vi "Synchronized Acquisition.vi"() -> ()   [LabVIEW 2018, in "GettingStarted_5775_Host.lvlib"]
uses:
  GettingStarted_5775_Host.lvlib
  <vilib>/userDefined/High Color/nirio_resource_hc.ctl
  <instrlib>/FlexRIO/API/Host/v1/NI FlexRIO/API/Reference Clock Source.ctl
  <vilib>/FPGAPlugInAG/Dynamic/niLvFpga_Reset_Dynamic.vi
  <vilib>/FPGAPlugInAG/Dynamic/niLvFpga_Run_Dynamic.vi
  <instrlib>/FlexRIO/API/Host/v1/NI FlexRIO/API/Configure Reference Clock.vi
  <instrlib>/FlexRIO/API/Host/v1/NI FlexRIO/API/Configure Immediate Start Trigger.vi
  <instrlib>/FlexRIO/API/Host/v1/NI FlexRIO/API/Configure Analog Start Trigger.vi
  <instrlib>/FlexRIO/API/Host/v1/NI FlexRIO/API/Configure Digital Edge Start Trigger.vi
  <instrlib>/FlexRIO/API/Host/v1/NI FlexRIO/API/Get Property Reference - Fpga Small.vi
  <instrlib>/FlexRIO/API/Host/v1/NI FlexRIO/API/Read Stream 1D WDT.vi
  <vilib>/FPGAPlugInAG/Dynamic/niLvFpga_Close_Dynamic.vi
  <vilib>/rvi/interface/nirviMethod/nirviMethod.xnode
  <vilib>/rvi/interface/nirviCloseFPGA/nirviCloseFPGA.xnode
  <instrlib>/FlexRIO/API/Host/v1/NI FlexRIO API v1.lvlib
  <resource>/objmgr/sessionReference.rc
  <resource>/objmgr/niflexrioapiStream.rc
panel:
  in  "reference clock source":T1 items=["Default", "Onboard", "PXI_Clk10", "External", "None", "Baseboard Reference"]
  in  "stop":bool
  out "error out":errorcluster
  out "Waveform Graph":waveform(dbl)[](graph)
  in  "acquire pretrigger \nsamples?":bool
  in  "min. TClk period":dbl=1e-06 format="%#_6p"
  in  "trigger master index":i32
  in  "Tab Control":enum32{"Immediate", "Digital", "Analog"}(tab)
  in  "trigger source":string(combo)="PXI_Trig0"
  in  "rising edge?":bool=TRUE
  in  "trigger channel":string="AI0"
  in  "level (V)":dbl
  in  "hysteresis (V)":dbl
  in  "device configuration":T3(array[cluster])=[{"FlexRIO digitizer"="RIO0", "channels"="AI0", "samples"=65536, "bitfile path"=path ""}, {"FlexRIO digitizer"="RIO1", "channels"="AI0", "samples"=65536, "bitfile path"=path ""}]
  # "Overview: Configure multiple FlexRIO targets for a synchronized acquisition using the FlexRIO Host API and NI-TClk API.\nRequirements: FlexRIO, NI-TClk\nInstructions: \n 1. Fill in the device configuration array with the resource name of the FlexRIO digitizers to synchronize, as well as the number of samples and which channels to acquire on.\n 2. Specify which device should be used as the trigger master using trigger master index\n 3. Configure the trigger settings for the master device\n 4. Optionally configure the reference clock to be used\n 5. Run the VI"
  # "Trigger Master Configuration"
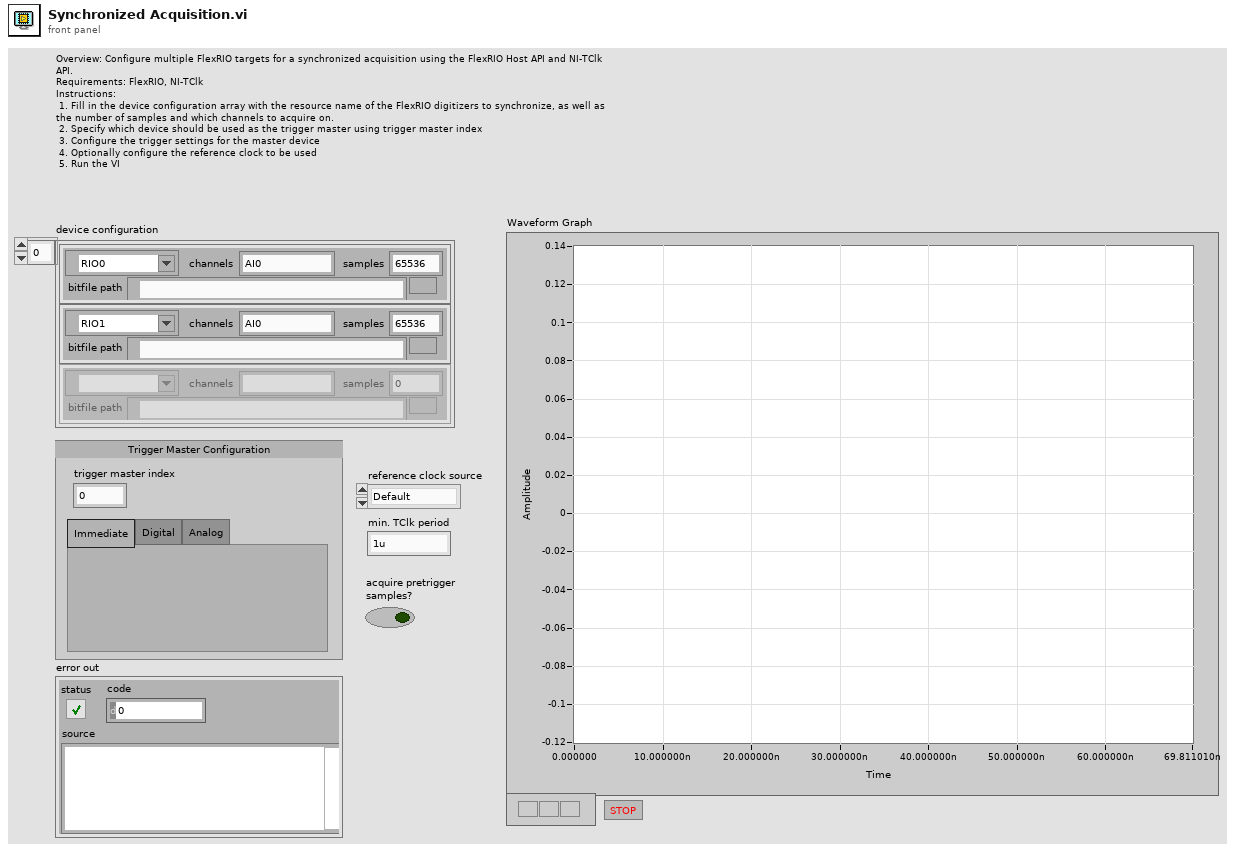
[diagram p1: front panel]
types:
  T1 = typedef "NI FlexRIO API v1.lvlib/Reference Clock Source.ctl" = i32
  T2 = typedef "nirio_resource_hc.ctl" = tag
  T3 = cluster{"FlexRIO digitizer":T2, "channels":string, "samples":u64, "bitfile path":path}[]
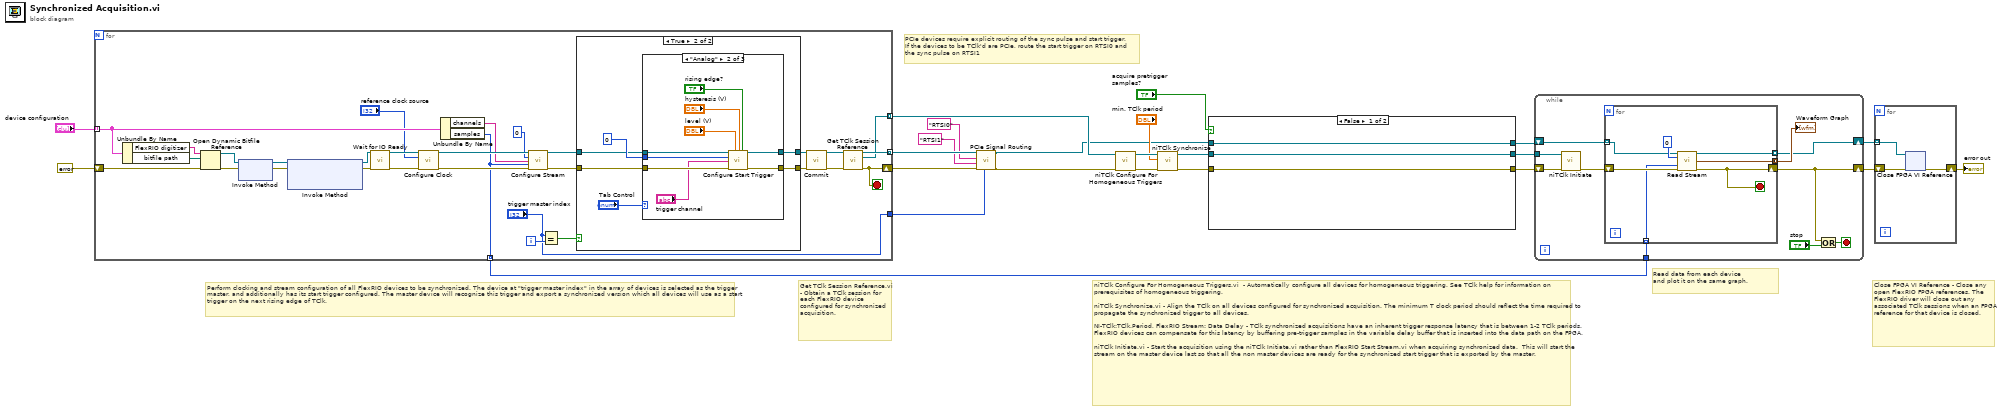
[diagram p0: block diagram]
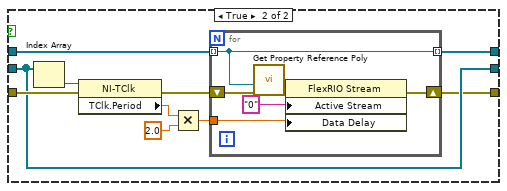
[diagram p2: hidden frame]
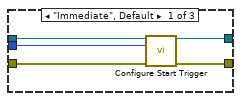
[diagram p4: hidden frame]
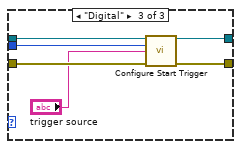
[diagram p5: hidden frame]
diagram:
  # "PCIe devices require explicit routing of the sync pulse and start trigger.\nIf the devices to be TClk'd are PCIe, route the start trigger on RTSI0 and\nthe sync pulse on RTSI1"
  # "Get TClk Session Reference.vi  - Obtain a TClk session for each FlexRIO device configured for synchronized acquisition."
  # "Perform clocking and stream configuration of all FlexRIO devices to be synchronized. The device at \"trigger master index\" in the array of devices is selected as the trigger master, and additionally has its start trigger configured. The master device will recognize this trigger and export a synchronized version which all devices will use as a start trigger on the next rising edge of TClk."
  # "niTClk Configure For Homogeneous Triggers.vi  - Automatically configure all devices for homogeneous triggering. See TClk help for information on prerequisites of homogeneous triggering. \n\nniTClk Synchronize.vi - Align the TClk on all devices configured for synchronized acquisition. The minimum T clock period should reflect the time required to propagate the synchronized trigger to all devices. \n\nNI-TClk:TClk.Period, FlexRIO Stream: Data Delay - TClk synchronized acquisitions have an inherent trigger response latency that is between 1-2 TClk periods. FlexRIO devices can compensate for this latency by buffering pre-trigger samples in the variable delay buffer that is inserted into the data path on the FPGA. \n\nniTClk Initiate.vi - Start the acquisition using the niTClk Initiate.vi rather than FlexRIO Start Stream.vi when acquiring synchronized data.  This will start the stream on the master device last so that all the non master devices are ready for the synchronized start trigger that is exported by the master."
  # "Read data from each device\nand plot it on the same graph."
  # "Close FPGA VI Reference - Close any open FlexRIO FPGA references. The FlexRIO driver will close out any associated TClk sessions when an FPGA reference for that device is closed."
  n1 = for {
    tunnel: "device configuration" -> [w47] mode=indexing
    tunnel: [w38] -> w6 mode=indexing
    tunnel: [w37] -> w11 mode=indexing
    shift-right: [w36] -> w7
    shift-left: errorcluster {"status"=FALSE, "code"=0, "source"=""} ("error out") -> [w27]
    tunnel: [w35] -> w14 mode=indexing
    tunnel: ["trigger master index"] -> w3
    i -> [w39]
    stop <- w36 stop-if-true
    n2 = Unbundle By Name(w47) -> ("FlexRIO digitizer"=w26:T2, "bitfile path"=w25:path)
    n3 = Open Dynamic Bitfile Reference(0:w26, 1:w25, 3:w27) -> (5:w24:refnum<k20>, 8:w28:errorcluster)  [unwired: 2 in]
    n4 = xnode "Invoke Method"("FPGA VI Reference In"=w24, "error in"=w28) -> ("FPGA VI Reference Out"=w32:refnum<k20>, "error out"=w33:errorcluster)
    n5 = xnode "Invoke Method"("FPGA VI Reference In"=w32, "error in"=w33) -> ("FPGA VI Reference Out"=w30:refnum<k20>, "error out"=w31:errorcluster)  [unwired: 1 in]
    n6 = call <instrlib>:"Wait for IO Ready.vi"("fpga interface in"=w30, "error in"=w31) -> ("fpga interface out"=w53:refnum<k20>, "error out"=w52:errorcluster)  [unwired: 10 in, 2 out]
    n7 = call-poly <instrlib>:"Configure Clock.vi"("fpga interface in"=w53, "reference clock source"="reference clock source", "error in"=w52) -> ("fpga interface out"=w51:refnum<k20>, "error out"=w50:errorcluster)  [unwired: 11 in]
    n8 = Unbundle By Name(w47) -> ("channels"=w46:string, "samples"=w35:u64)
    n9 = call <instrlib>:"Configure Stream.vi"("fpga interface in"=w51, "stream instance"=u32 0, "channels enabled"=w46, "num samples"=w35, "error in"=w50) -> ("fpga interface out"=w48:refnum<k20>, "error out"=w49:errorcluster)  [unwired: 7 in, 2 out]
    n10 = Equal?(x="trigger master index", y=w39) -> (x = y?=w40:bool)
    n11 = case shown="True" w40 {
      tunnel: w49 -> [w54 w59]
      tunnel: w48 -> [w55 w58]
      tunnel: [w54 w57] -> w44
      tunnel: [w55 w56] -> w43
      frame False {
      }
      frame True {
        n12 = case shown="\"Analog\"" "Tab Control" {
          tunnel: w59 -> [w66 w75 w81]
          tunnel: [w65 w74 w80] -> w57
          tunnel: w58 -> [w64 w73 w79]
          tunnel: [w63 w72 w78] -> w56
          tunnel: u32 0 -> [w62 w71 w77]
          frame "Immediate", Default {
            n13 = call-poly <instrlib>:"Configure Start Trigger.vi"("fpga interface in"=w64, "trigger instance"=w62, "error in"=w66) -> ("fpga interface out"=w63:refnum<k20>, "error out"=w65:errorcluster)  [unwired: 10 in, 1 out]
          }
          frame "Analog" {
            n14 = call-poly <instrlib>:"Configure Start Trigger.vi"("fpga interface in"=w73, "level"="level (V)", "hysteresis"="hysteresis (V)", "rising edge?"="rising edge?", "trigger instance"=w71, "channel"="trigger channel", "error in"=w75) -> ("fpga interface out"=w72:refnum<k20>, "error out"=w74:errorcluster)  [unwired: 6 in, 1 out]
          }
          frame "Digital" {
            n15 = call-poly <instrlib>:"Configure Start Trigger.vi"("fpga interface in"=w79, "trigger instance"=w77, "trigger source"="trigger source", "error in"=w81) -> ("fpga interface out"=w78:refnum<k20>, "error out"=w80:errorcluster)  [unwired: 9 in, 1 out]
          }
        }
      }
    }
    n16 = call <instrlib>:"Commit.vi"("fpga interface in"=w43, "error in"=w44) -> ("fpga interface out"=w42:refnum<k20>, "error out"=w41:errorcluster)  [unwired: 12 in]
    n17 = call <instrlib>:"Get TClk Session Reference.vi"("fpga interface in"=w42, "error in"=w41) -> ("fpga interface out"=w38:refnum<k20>, "tclk session reference"=w37:refnum<k20>, "error out"=w36:errorcluster)  [unwired: 11 in]
  }
  n18 = call "PCIe Signal Routing.vi"("trigger master index"=w3, "error in"=w7, "sync pulse rtsi line"="RTSI1", "start trigger rtsi line"="RTSI0", "fpga interfaces in"=w6) -> ("error out"=w1:errorcluster, "fpga interfaces out"=w2:refnum<k20>[])  [unwired: 5 in]
  n19 = call <instrlib>:"niTClk Configure For Homogeneous Triggers.vi"("error in (no error)"=w1, "sessions"=w11) -> ("error out"=w22:errorcluster, "sessions out"=w21:refnum<k20>[])  [unwired: 8 in]
  n20 = call <instrlib>:"niTClk Synchronize.vi"("error in (no error)"=w22, "minimum T clock period"="min. TClk period", "sessions"=w21) -> ("error out"=w20:errorcluster, "sessions out"=w19:refnum<k20>[])  [unwired: 7 in]
  n21 = case shown="False" "acquire pretrigger \nsamples?" {
    tunnel: w2 -> [w84 w93]
    tunnel: [w84 w92] -> w9
    tunnel: w20 -> [w82 w91]
    tunnel: w19 -> [w83 w87]
    tunnel: [w83 w87] -> w10
    tunnel: [w82 w86] -> w18
    frame False {
    }
    frame True {
      n22 = Index Array(array=w87) -> (element=w94:refnum<k20>)  [unwired: 1 in]
      n23 = property class="NI-TClk"(reference=w94, error in=w91) -> (error out=w85:errorcluster, "TClk.Period"=w89:dbl)  [unwired: 1 out]
      n24 = Multiply(x=w89, y=2.0) -> (x*y=w88:dbl)
      n25 = for {
        tunnel: w93 -> [w95] mode=indexing
        tunnel: [w95] -> w92 mode=indexing
        tunnel: w88 -> [w99]
        shift-right: [w98] -> w86
        shift-left: w85 -> [w97]
        n26 = call-poly <instrlib>:"Get Property Reference Poly.vi"("error in (no error)"=w97, "fpga interface in"=w95) -> ("error out"=w96:errorcluster, "property reference"=w101:refnum<k20>)  [unwired: 4 in, 1 out]
        n27 = property class="FlexRIO Stream"(reference=w101, error in=w96, "Active Stream"="0", "Data Delay"=w99) -> (error out=w98:errorcluster)  [unwired: 1 out]
      }
    }
  }
  n28 = while {
    tunnel: w10 -> [w111]
    tunnel: w14 -> [w107]
    shift-right: [w102] -> w13
    shift-left: w18 -> [w110]
    shift-right: [w105] -> w8
    shift-left: w9 -> [w109]
    stop <- w104 stop-if-true
    n29 = call <instrlib>:"niTClk Initiate.vi"("error in (no error)"=w110, "sessions"=w111) -> ("error out"=w108:errorcluster)  [unwired: 8 in, 1 out]
    n30 = for {
      tunnel: w109 -> [w116] mode=indexing
      shift-right: [w112] -> w102
      shift-left: w108 -> [w117]
      tunnel: w107 -> [w115] mode=indexing
      tunnel: [w114] -> w105 mode=indexing
      tunnel: [w113] -> w106 mode=concatenating
      stop <- w112 stop-if-true
      n31 = call-poly <instrlib>:"Read Stream.vi"("fpga interface in"=w116, "stream instance"=u32 0 ("stream number"), "samples"=w115, "error in"=w117) -> ("fpga interface out"=w114:refnum<k20>, "read data"=w113:waveform(dbl)[], "error out"=w112:errorcluster)  [unwired: 7 in, 2 out]
    }
    "Waveform Graph" <- w106
    n32 = Or(x=w102, y="stop") -> (x .or. y?=w104:bool)
  }
  n33 = for {
    tunnel: w8 -> [w120] mode=indexing
    shift-right: [w119] -> w12
    shift-left: w13 -> [w121]
    n34 = xnode "Close FPGA VI Reference"("FPGA VI Reference In"=w120, "error in"=w121) -> ("error out"=w119:errorcluster)
  }
  "error out" <- w12
